vi "General Auto PID Simulator.vi"() -> ()   [LabVIEW 2023]
doc: "This example demonstrates how to simulate a simple control loop and a general plant model. This VI also demonstrates how you can use the PID Control VIs to autotune the PID gains."
uses:
  <vilib>/addons/control/pid/NI_PID_autopid.lvlib
panel:
  out "Controller Output":dbl(graph)
  in  "reinitialize? (F)":bool
  in  "Autotune":bool
  in  "PID gains":T1={"proportional gain (Kc)"=20.0, "integral time (Ti, min)"=0.008, "derivative time (Td, min)"=0.001} {"derivative time (Td, min)" format="%.3f"; "integral time (Ti, min)" format="%.3f"; "proportional gain (Kc)" format="%.3f"}
  in  "Sampling Time dt (s)":dbl=0.05 min=0.001 step=0.01 format="%#.3p"
  out "Output (+/- %)":dbl(slide)=100.0 scale=-100.0..100.0
  out "PV(%)":dbl(slide)=19.49158795728343 scale=0.0..100.0
  in  "Stop":bool
  in  "SP(%)":dbl(slide)=34.59119496855346 scale=0.0..100.0
  out "Process Variable and Setpoint":cluster{"initial PV":dbl, "SP(%)":dbl}(graph)
  # "Overview: This example demonstrates how to simulate a simple control loop and a general plant model.  This VI also demonstrates how you can use the PID Control VIs to autotune the PID gains.\nInstructions:\n1. Run the VI. When the PV value equals the SP value, click the Autotune button and follow the instructions in the PID Autotuning Wizard.\n2. Click Stop to stop the VI."
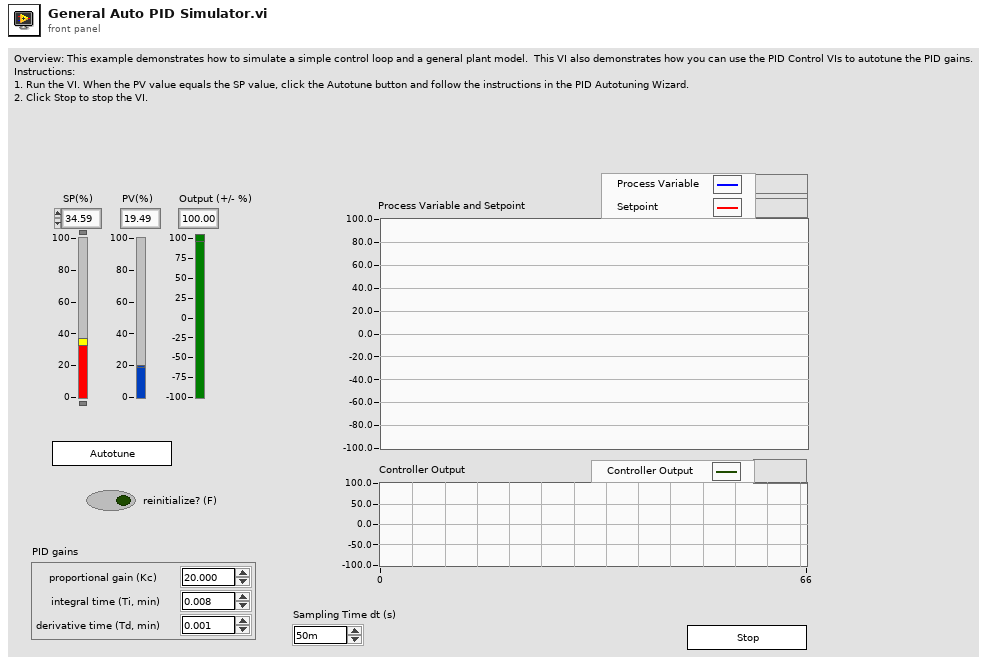
[diagram p1: front panel]
types:
  T1 = cluster{"proportional gain (Kc)":dbl, "integral time (Ti, min)":dbl, "derivative time (Td, min)":dbl}
  T2 = cluster{"static gain":dbl, "lag (min)":dbl, "dead cycles":i32, "load %":dbl, "deadband":dbl, "noise level %":dbl, "initial PV":dbl}
  T3 = cluster{"controller type":u16, "relay cycles":i32, "relay amplitude":dbl, "control specification":u16, "PV noise level":dbl}
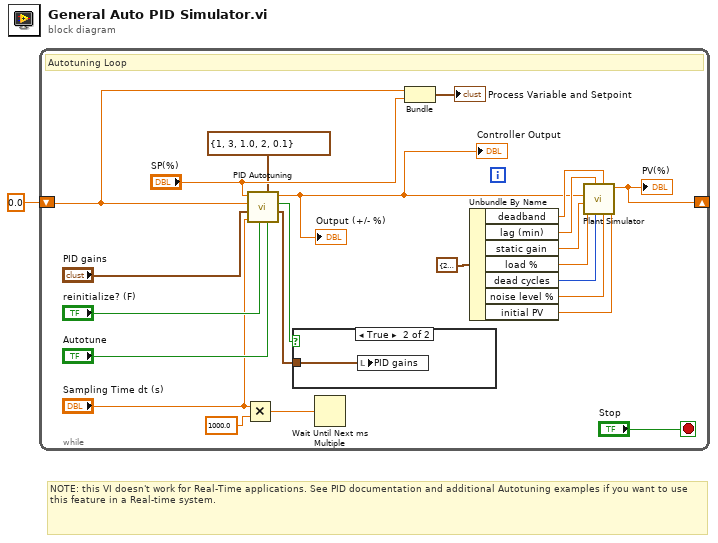
[diagram p0: block diagram]
diagram:
  # "NOTE: this VI doesn't work for Real-Time applications. See PID documentation and additional Autotuning examples if you want to use this feature in a Real-time system."
  n1 = while {
    shift-left: 0.0 ("Process Variable (%)") -> [w11]
    shift-right: [w13] -> _
    stop <- "Stop" stop-if-true
    # "Autotuning Loop"
    n2 = Multiply(x="Sampling Time dt (s)", y=1000.0) -> (x*y=w2:dbl)
    n3 = call <vilib>:"PID Autotuning.vi"("autotune? (F)"="Autotune", "autotuning parameters"=T3 {"controller type"=1, "relay cycles"=3, "relay amplitude"=1.0, "control specification"=2, "PV noise level"=0.1} ("autotuning initial parameters"), "reinitialize? (F)"="reinitialize? (F)", "dt (s)"="Sampling Time dt (s)", "PID gains"="PID gains", "process variable"=w11, "setpoint"="SP(%)") -> ("PID gains out"=w9:T1, "tuning completed?"=w8:bool, "output"=w3:dbl)  [unwired: 1 in, 1 out]
    "Output (+/- %)" <- w3
    "Controller Output" <- w3
    n4 = case shown="True" w8 {
      tunnel: w9 -> [_ w25]
      frame False {
      }
      frame True {
        n5 = local write "PID gains"(w25) -> ()
      }
    }
    n6 = Wait Until Next ms Multiple(millisecond multiple=w2) -> ()  [unwired: 1 out]
    n7 = Bundle("Process Variable (%)"=w11, "SP(%)"="SP(%)") -> (→"Process Variable and Setpoint":cluster{"Process Variable (%)":dbl, "SP(%)":dbl})  [unwired: 1 in]
    n8 = Unbundle By Name(T2 {"static gain"=2.5, "lag (min)"=0.3, "dead cycles"=1, "load %"=40.0, "deadband"=2.0, "noise level %"=0.25, "initial PV"=0.0} ("process parameters")) -> ("deadband"=w20:dbl, "lag (min)"=w14:dbl, "static gain"=w19:dbl, "load %"=w18:dbl, "dead cycles"=w22:i32, "noise level %"=w15:dbl, "initial PV"=w12:dbl)
    n9 = call "Plant Simulator.vi"("Initial PV"=w12, "Controller Noise (%)"=w15, "Valve Deadband"=w20, "Process Deadtime"=w22, "Lag (min)"=w14, "Process Load"=w18, "Process Gain"=w19, "Manipulated Variable (Output, %)"=w3) -> ("Process Variable (%)"=w13:dbl)  [unwired: 3 in]
    "PV(%)" <- w13
  }
